vi "Logger_GetDatePathAndDataName.vi"(8 "error in (no error)":errorcluster caption="错误输入（无错误）", 11 "Logger 输入":refnum<class "Logger.lvclass">) -> (0 "error out":errorcluster caption="错误输出", 1 "dataname":string, 2 "datepath":string, 3 "Logger 输出":refnum<class "Logger.lvclass">)   [LabVIEW 2019, in "Logger.lvclass"]
uses:
  <userlib>/Logger/Logger.lvclass
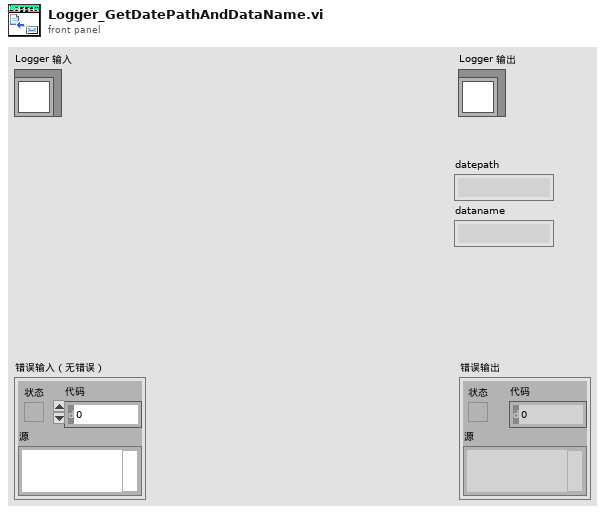
[diagram p1: front panel]
types:
  T1 = typedef "Logger.lvclass/LoggerSaveTime.ctl" = enum16{"每小时保存", "每天保存", "每周保存", "每月保存"}
  T2 = typedef "LVDateTimeRec.ctl" = cluster{"秒数的小数部分":dbl, "秒":i32, "分":i32, "时":i32, "日":i32, "月":i32, "年":i32, "天数（周）":i32, "天数（年）":i32, "DST":i32}
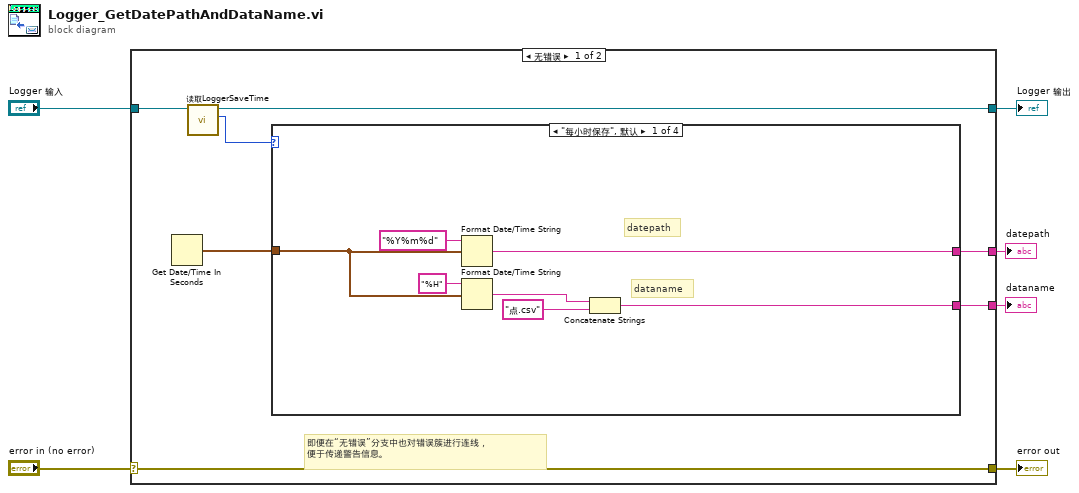
[diagram p0: block diagram]
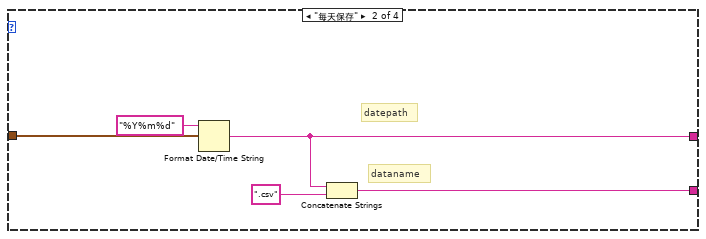
[diagram p2: hidden frame]
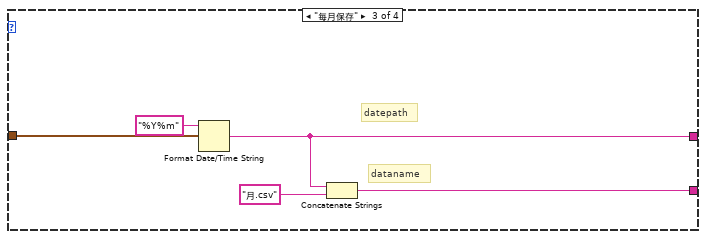
[diagram p3: hidden frame]
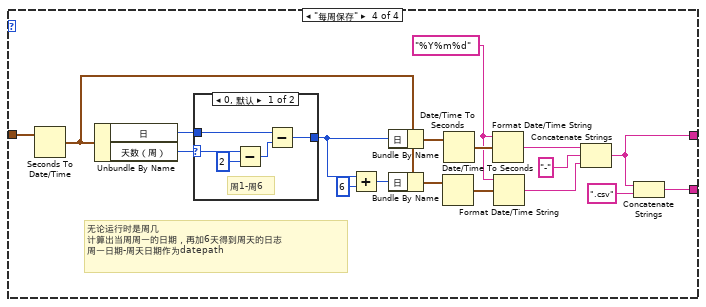
[diagram p4: hidden frame]
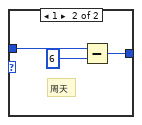
[diagram p5: hidden frame]
diagram:
  n1 = case shown="无错误" "error in (no error)" {
    selector: "error in (no error)" -> [w13 w58]
    tunnel: [w13 w58] -> w5
    tunnel: [w11 w57] -> w3
    tunnel: "Logger 输入" -> [w12 w57]
    tunnel: [w8 _] -> w2
    tunnel: [w7 _] -> w1
    frame No Error {
      # "即便在“无错误”分支中也对错误簇进行连线，\n便于传递警告信息。"
      n2 = Get Date/Time In Seconds() -> (seconds since 1Jan1904=w9:timestamp)
      n3 = call "读取LoggerSaveTime.vi"("Logger输入"=w12) -> ("LoggerSaveTime"=w10:T1, "Logger输出"=w11:refnum<class "Logger.lvclass">)  [unwired: 8 in, 1 out]
      n4 = case shown="\"每小时保存\", 默认" w10 {
        tunnel: w9 -> [w15 w22 w27 w35]
        tunnel: [w19 w21 w26 w32] -> w8
        tunnel: [w17 w23 w28 w33] -> w7
        frame "每小时保存", Default {
          # "dataname"
          # "datepath"
          n5 = Format Date/Time String(time format string (%c)="%Y%m%d" ("时间格式字符串(%c)"), seconds (now)=w15) -> (date/time string=w19:string)  [unwired: 1 in]
          n6 = Format Date/Time String(time format string (%c)="%H" ("时间格式字符串(%c)"), seconds (now)=w15) -> (date/time string=w14:string)  [unwired: 1 in]
          n7 = Concatenate Strings(w14, "点.csv" ("字符串")) -> (w17:string)
        }
        frame "每天保存" {
          # "dataname"
          # "datepath"
          n8 = Format Date/Time String(time format string (%c)="%Y%m%d" ("时间格式字符串(%c)"), seconds (now)=w22) -> (date/time string=w21:string)  [unwired: 1 in]
          n9 = Concatenate Strings(w21, ".csv" ("字符串")) -> (w23:string)
        }
        frame "每月保存" {
          # "dataname"
          # "datepath"
          n10 = Format Date/Time String(time format string (%c)="%Y%m" ("时间格式字符串(%c)"), seconds (now)=w27) -> (date/time string=w26:string)  [unwired: 1 in]
          n11 = Concatenate Strings(w26, "月.csv" ("字符串")) -> (w28:string)
        }
        frame "每周保存" {
          w36 = "%Y%m%d" ("时间格式字符串(%c)")
          # "无论运行时是周几\n计算出当周周一的日期，再加6天得到周天的日志\n周一日期-周天日期作为datepath"
          n12 = Seconds To Date/Time(time stamp (now)=w35) -> (date time rec=w34:T2)  [unwired: 1 in]
          n13 = Unbundle By Name(w34) -> ("日"=w47:i32, "天数（周）"=w48:i32)
          n14 = case shown="0, 默认" w48 {
            selector: w48 -> [w52 _]
            tunnel: w47 -> [w51 w56]
            tunnel: [w49 w54] -> w43
            frame 0, Default {
              # "周1-周6"
              n15 = Subtract(x=w52, y=2) -> (x-y=w50:i32)
              n16 = Subtract(x=w51, y=w50) -> (x-y=w49:i32)
            }
            frame 1 {
              # "周天"
              n17 = Subtract(x=w56, y=6) -> (x-y=w54:i32)
            }
          }
          n18 = Add(x=w43, y=6) -> (x+y=w44:i32)
          n19 = Bundle By Name(cluster=w34, "日"=w43) -> (w45:T2)
          n20 = Bundle By Name(cluster=w34, "日"=w44) -> (w40:T2)
          n21 = Date/Time To Seconds(2:w40) -> (0:w41:timestamp)  [unwired: 1 in]
          n22 = Date/Time To Seconds(2:w45) -> (0:w46:timestamp)  [unwired: 1 in]
          n23 = Format Date/Time String(time format string (%c)=w36, seconds (now)=w46) -> (date/time string=w39:string)  [unwired: 1 in]
          n24 = Format Date/Time String(time format string (%c)=w36, seconds (now)=w41) -> (date/time string=w38:string)  [unwired: 1 in]
          n25 = Concatenate Strings(w39, "-" ("字符串"), w38) -> (w32:string)
          n26 = Concatenate Strings(w32, ".csv" ("字符串")) -> (w33:string)
        }
      }
    }
    frame Error {
    }
  }
  "error out" <- w5
  "Logger 输出" <- w3
  "datepath" <- w2
  "dataname" <- w1
